vi "CRYStepData Manipulate.vi"(7 "sAction":string, 10 "StepNo.":i32) -> ()   [LabVIEW 2013]
uses:
  Global/CRYCurves Array Global.vi
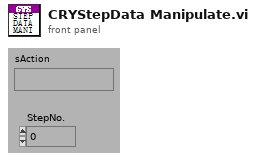
[diagram p1: front panel]
types:
  T1 = typedef "CRYWaveform Cluster Array.ctl" = T2[]
  T2 = typedef "CRYWaveform Cluster.ctl" = cluster{"Waveform":cluster{"X0":dbl, "dX":dbl, "Y":sgl[]}, "X data":u16, "Y data":u16, "Y axis":u16, "X unit":string, "Y unit":string, "Y dB ref":dbl, "display Y":bool, "display X":bool, "Overload?":bool, "Test Info":string, "Step No.":i32, "Name":string, "protected":bool, "Sqc history":string[], "Signal Channel ID":i32, "Plot Settings":cluster{"Color":u32, "Interpolation":u8, "Point Style":u8, "Line Style":u8, "Point Color":u32, "Line Width":u8, "Bar Plot Style":u8, "Fill To":i16}, "AutoProtect":bool}
  T3 = typedef "CRYResult Cluster Array.ctl" = T4[]
  T4 = typedef "CRYResult Cluster.ctl" = cluster{"Name":string, "Margin":dbl, "unit":string, "Verdict":bool, "Limit":string, "Max/Min":string, "protected":bool, "Step No.":i32, "Test Info":string, "AutoProtect":bool}
  T5 = typedef "CRYData Cluster Array.ctl" = T6[]
  T6 = typedef "CRYData Cluster.ctl" = cluster{"Name":string, "Curve":cluster{"x":dbl, "y":dbl, "z":dbl}[], "X data":u16, "Y data":u16, "Z data":u16, "X axis":u16, "Y axis":u16, "Z axis":u16, "X unit":string, "Y unit":string, "Z unit":string, "X dB ref":dbl, "Y dB ref":dbl, "Z dB ref":dbl, "single val":bool, "protected":bool, "display X":bool, "display Y":bool, "display Z":bool, "Test Info":string, "Step No.":i32, "Plot Settings":cluster{"Color":u32, "Interpolation":u8, "Point Style":u8, "Line Style":u8, "Point Color":u32, "Line Width":u8, "Bar Plot Style":u8, "Fill To":i16}, "AutoProtect":bool}
  T7 = typedef "CRYStep.ctl" = cluster{"No.VI":i32, "Category":string, "StepName":string, "Seq setup flattened":string, "Comment":string, "Steps config.":bool[], "Jump config":i32[], "Start":dbl, "Increment":dbl, "Name":string, "Unit":string, "Y data":u16, "Y prefix":string, "Y dB ref":dbl, "Y unit":string, "Repeat State Array":cluster{"Start":dbl, "Increment":dbl, "Count":i32, "Num":i32}[]}
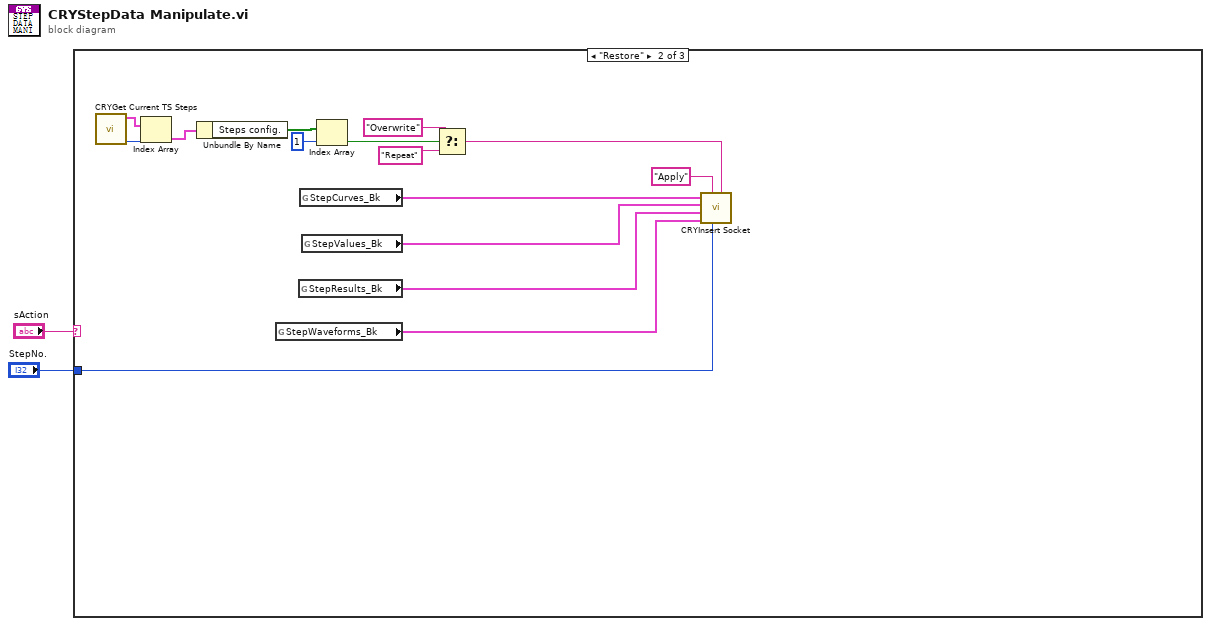
[diagram p0: block diagram]
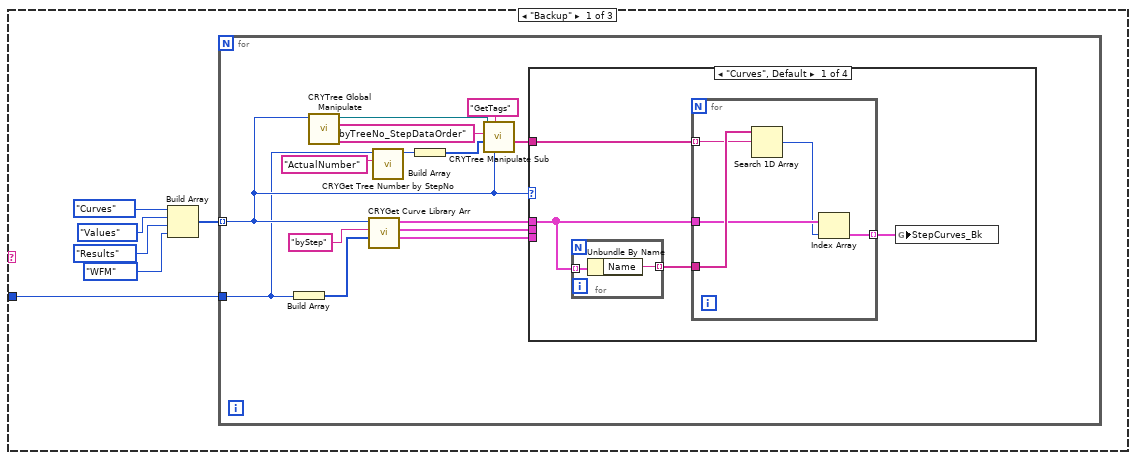
[diagram p2: hidden frame]
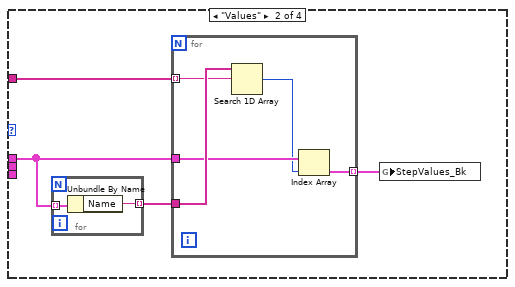
[diagram p3: hidden frame]
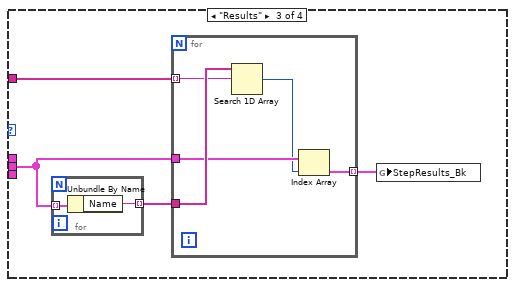
[diagram p4: hidden frame]
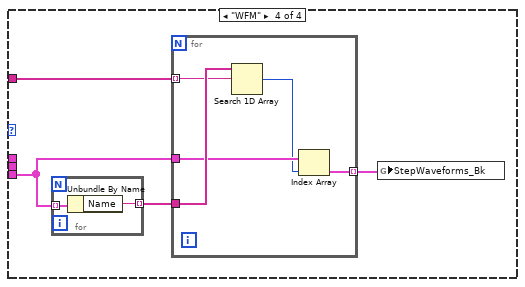
[diagram p5: hidden frame]
diagram:
  n1 = case shown="\"Restore\"" "sAction" {
    tunnel: "StepNo." -> [w3 w76 _]
    frame "Backup" {
      n2 = Build Array(enum16{"Curves", "Values", "Results", "WFM"}."Curves" ("Type"), enum16{"Curves", "Values", "Results", "WFM"}."Values" ("Type"), enum16{"Curves", "Values", "Results", "WFM"}."Results" ("Type"), enum16{"Curves", "Values", "Results", "WFM"}."WFM" ("Type")) -> (w4:enum16{"Curves", "Values", "Results", "WFM"}[])
      n3 = for {
        tunnel: w4 -> [w17] mode=indexing
        tunnel: w3 -> [w11]
        n4 = Build Array(w11) -> (w12:i32[])
        n5 = call "CRYTree Global Manipulate.vi"("Type In"=w17) -> ("Tree/Curve Tree"=w18:refnum<vi>)  [unwired: 7 in, 3 out]
        n6 = call "CRYGet Curve Library Arr.vi"("Index"=w12, "sOption"="byStep", "Type In"=w17) -> ("Waveforms"=w19:T1, "Results"=w20:T3, "Curves/Values"=w21:T5)  [unwired: 6 in]
        n7 = call "CRYGet Tree Number by StepNo.vi"("sOption"="ActualNumber", "Step Setup VI No"=w11) -> ("Number in Tree"=w10:i32)  [unwired: 8 in, 1 out]
        n8 = Build Array(w10) -> (w9:i32[])
        n9 = call "CRYTree Manipulate Sub.vi"("Type"=w17, "sAction"="GetTags", "nData"=w9, "sOption"="byTreeNo_StepDataOrder", "Tree in"=w18) -> ("sData Out"=w14:string[])  [unwired: 2 in, 4 out]
        n10 = case shown="\"Curves\", Default" w17 {
          tunnel: w21 -> [w25 w36 _ _]
          tunnel: w20 -> [_ _ w46 _]
          tunnel: w19 -> [_ _ _ w56]
          tunnel: w14 -> [w26 w37 w48 w59]
          frame "Curves", Default {
            n11 = for {
              tunnel: w25 -> [w28] mode=indexing
              tunnel: [w27] -> w24 mode=indexing
              n12 = Unbundle By Name(w28) -> ("Name"=w27:string)
            }
            n13 = for {
              tunnel: w25 -> [w31]
              tunnel: w26 -> [w32] mode=indexing
              tunnel: w24 -> [w33]
              tunnel: [w29] -> w23 mode=indexing
              n14 = Search 1D Array(1D array=w33, element=w32) -> (index of element=w30:i32)  [unwired: 1 in]
              n15 = Index Array(array=w31, index=w30) -> (element=w29:T6)
            }
            n16 = global write "CRYCurves Array Global.vi" "StepCurves_Bk"(w23) -> ()
          }
          frame "Values" {
            n17 = for {
              tunnel: w36 -> [w39] mode=indexing
              tunnel: [w38] -> w35 mode=indexing
              n18 = Unbundle By Name(w39) -> ("Name"=w38:string)
            }
            n19 = for {
              tunnel: w36 -> [w42]
              tunnel: w37 -> [w43] mode=indexing
              tunnel: w35 -> [w44]
              tunnel: [w40] -> w34 mode=indexing
              n20 = Search 1D Array(1D array=w44, element=w43) -> (index of element=w41:i32)  [unwired: 1 in]
              n21 = Index Array(array=w42, index=w41) -> (element=w40:T6)
            }
            n22 = global write "CRYCurves Array Global.vi" "StepValues_Bk"(w34) -> ()
          }
          frame "Results" {
            n23 = for {
              tunnel: w46 -> [w50] mode=indexing
              tunnel: [w49] -> w47 mode=indexing
              n24 = Unbundle By Name(w50) -> ("Name"=w49:string)
            }
            n25 = for {
              tunnel: w46 -> [w53]
              tunnel: w48 -> [w54] mode=indexing
              tunnel: w47 -> [w55]
              tunnel: [w51] -> w45 mode=indexing
              n26 = Search 1D Array(1D array=w55, element=w54) -> (index of element=w52:i32)  [unwired: 1 in]
              n27 = Index Array(array=w53, index=w52) -> (element=w51:T4)
            }
            n28 = global write "CRYCurves Array Global.vi" "StepResults_Bk"(w45) -> ()
          }
          frame "WFM" {
            n29 = for {
              tunnel: w56 -> [w61] mode=indexing
              tunnel: [w60] -> w58 mode=indexing
              n30 = Unbundle By Name(w61) -> ("Name"=w60:string)
            }
            n31 = for {
              tunnel: w56 -> [w64]
              tunnel: w59 -> [w65] mode=indexing
              tunnel: w58 -> [w66]
              tunnel: [w62] -> w57 mode=indexing
              n32 = Search 1D Array(1D array=w66, element=w65) -> (index of element=w63:i32)  [unwired: 1 in]
              n33 = Index Array(array=w64, index=w63) -> (element=w62:T2)
            }
            n34 = global write "CRYCurves Array Global.vi" "StepWaveforms_Bk"(w57) -> ()
          }
        }
      }
    }
    frame "Restore" {
      n35 = call "CRYGet Current TS Steps.vi"() -> ("SelectStepNumber in Tree"=w74:i32, "Steps"=w75:T7[])  [unwired: 1 in, 9 out]
      n36 = Index Array(array=w75, index=w74) -> (element=w73:T7)
      n37 = Unbundle By Name(w73) -> ("Steps config."=w72:bool[])
      n38 = global read "CRYCurves Array Global.vi" "StepWaveforms_Bk"() -> (w68:T1)
      n39 = global read "CRYCurves Array Global.vi" "StepResults_Bk"() -> (w69:T3)
      n40 = global read "CRYCurves Array Global.vi" "StepCurves_Bk"() -> (w71:T5)
      n41 = global read "CRYCurves Array Global.vi" "StepValues_Bk"() -> (w70:T5)
      n42 = Index Array(array=w72, index=1) -> (element=w78:bool)
      n43 = Select(t="Overwrite" ("Y unit"), s=w78, f="Repeat") -> (s? t:f=w77:string)
      n44 = call "CRYInsert Socket.vi"("sOption2"=w77, "Step No."=w76, "sOption1"="Apply", "Waves"=w68, "Results"=w69, "Values"=w70, "Curves"=w71) -> ()  [unwired: 4 in, 1 out]
    }
    frame Default {
    }
  }
